vi "get columns.vi"(9 "columns  INFO":string[](array[string]), 10 "columns外部输入":T1, 11 "数组":variant[][](array[variant])) -> (2 "columns output":string[](array[string]), 3 "data":string[][](array[string]))   [LabVIEW 2016, in "SQLite Lib.lvlib"]
uses:
  SQLite Lib.lvlib
  <vilib>/Utility/VariantDataType/VariantType.lvlib
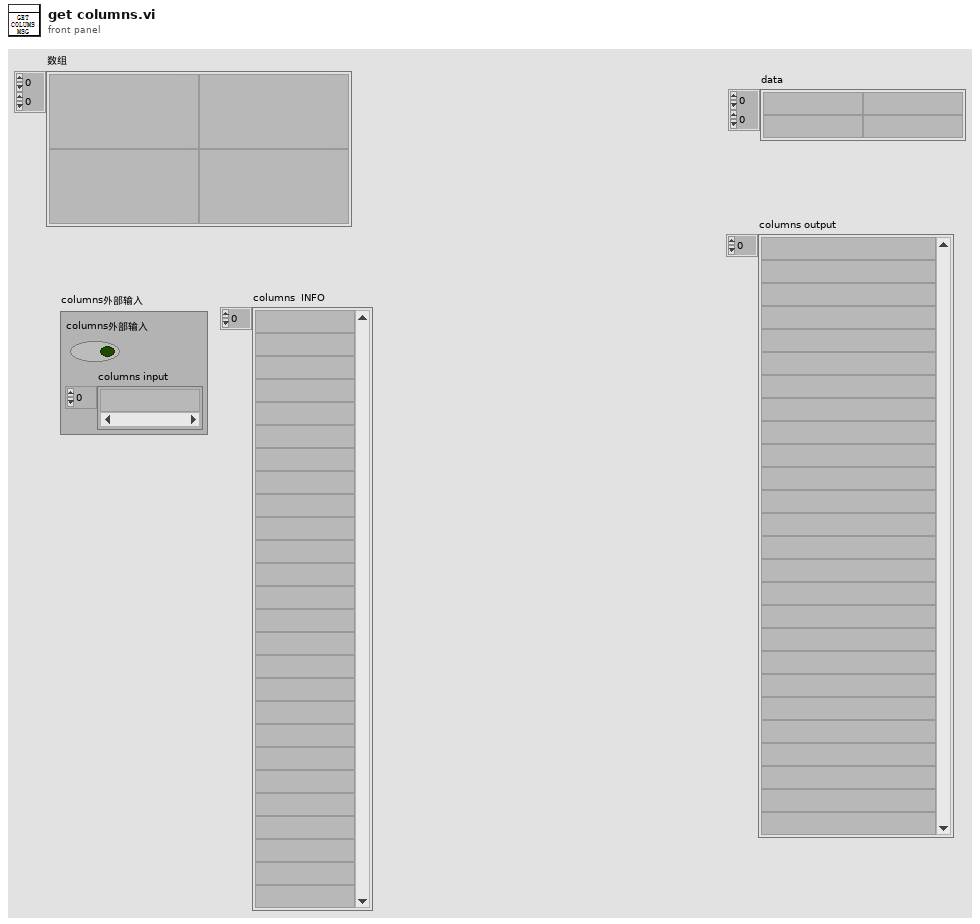
[diagram p1: front panel]
types:
  T1 = cluster{"columns外部输入":bool, "columns input":string[]}
  T2 = typedef "VariantType.lvlib/Type.ctl" = enum8{"Invalid Type", "Void", "I8", "I16", "I32", "I64", "U8", "U16", "U32", "U64", "Single Float", "Double Float", "Extended Float", "Single Complex", "Double Complex", "Extended Complex", "Enum U8", "Enum U16", "Enum U32", "Enum U64", "Single Float With Unit", "Double Float With Unit", "Extended Float With Unit", "Single Complex with Unit", "Double Complex with Unit", "Extended Complex with Unit", "Boolean", "String", "Path", "Picture", "Tag", "Array", "Cluster", "Variant", "LV Variant", "Waveform", "Timestamp", "Digital Waveform", "Digital Data", "ExpressData", "Refnum", "External Data", "VI", "Poly VI", "LabVIEW Class Instance", "Fixed Point"}
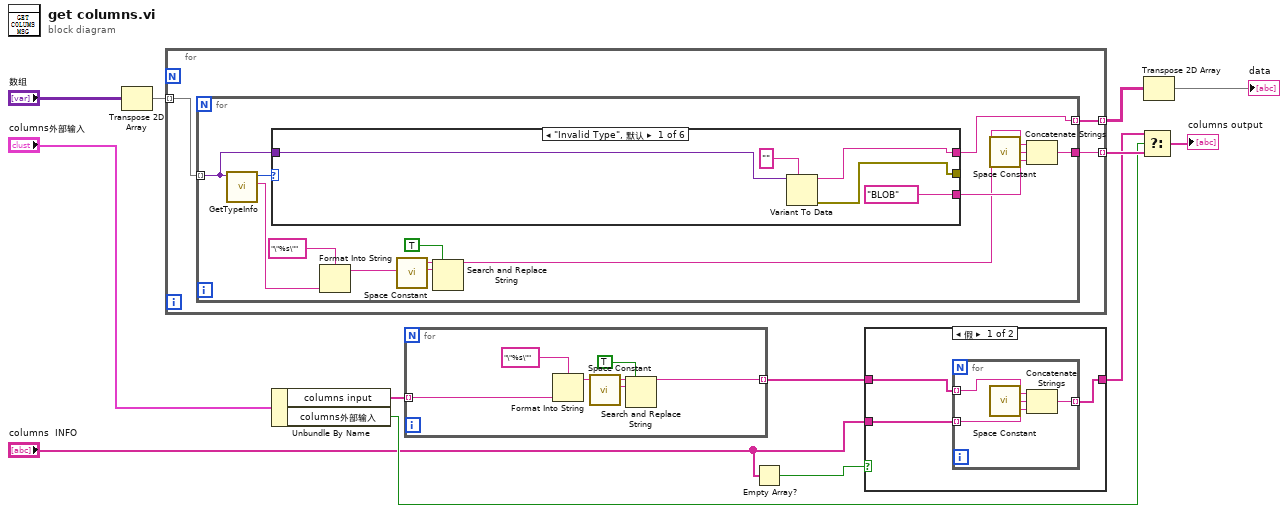
[diagram p0: block diagram]
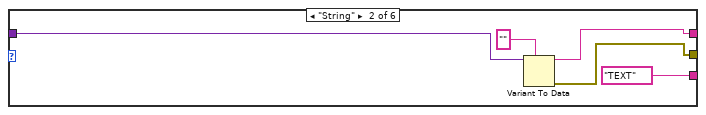
[diagram p3: hidden frame]
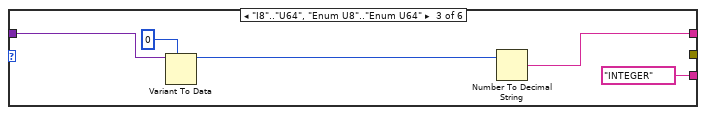
[diagram p4: hidden frame]
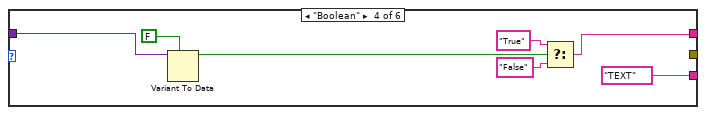
[diagram p5: hidden frame]
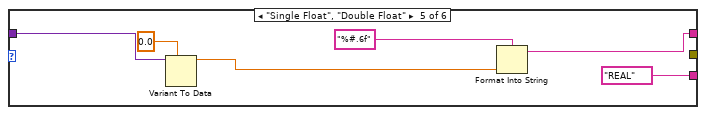
[diagram p6: hidden frame]
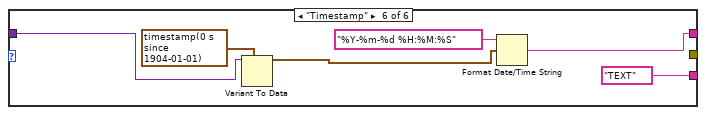
[diagram p7: hidden frame]
diagram:
  n1 = Transpose 2D Array(2D array="数组") -> (transposed array=w11:variant[][])
  n2 = for {
    tunnel: [w14] -> w9 mode=indexing
    tunnel: [w16] -> w12 mode=indexing
    tunnel: w11 -> [w15] mode=indexing
    n3 = for {
      tunnel: [w28] -> w16 mode=indexing
      tunnel: w15 -> [w27] mode=indexing
      tunnel: [w26] -> w14
      n4 = call <vilib>:"GetTypeInfo.vi"("Variant"=w27) -> ("Name"=w21:string, "Type Enum"=w23:T2)  [unwired: 6 in, 3 out]
      n5 = case shown="\"Invalid Type\", 默认" w23 {
        tunnel: w27 -> [w33 w38 w43 w50 w56 w62]
        tunnel: [w31 w36 w40 w44 w53 w59] -> w28
        tunnel: [w30 w35 _ _ _ _] -> _
        tunnel: ["BLOB" ("组合框") "TEXT" ("组合框") "INTEGER" ("组合框") "TEXT" ("组合框") "REAL" ("组合框") "TEXT" ("组合框")] -> w25
        frame "Invalid Type", Default {
          n6 = Variant To Data(type="", Variant=w33) -> (data=w31:string, error out=w30:errorcluster)  [unwired: 1 in]
        }
        frame "String" {
          n7 = Variant To Data(type="", Variant=w38) -> (data=w36:string, error out=w35:errorcluster)  [unwired: 1 in]
        }
        frame "I8".."U64", "Enum U8".."Enum U64" {
          n8 = Variant To Data(type=0, Variant=w43) -> (data=w41:i32)  [unwired: 1 in, 1 out]
          n9 = Number To Decimal String(number=w41) -> (decimal integer string=w40:string)  [unwired: 1 in]
        }
        frame "Boolean" {
          n10 = Variant To Data(type=FALSE, Variant=w50) -> (data=w47:bool)  [unwired: 1 in, 1 out]
          n11 = Select(t="True", s=w47, f="False") -> (s? t:f=w44:string)
        }
        frame "Single Float", "Double Float" {
          n12 = Variant To Data(type=sgl 0.0, Variant=w56) -> (data=w54:sgl)  [unwired: 1 in, 1 out]
          n13 = Format Into String(format string="%#.6f" ("格式字符串"), w54) -> (resulting string=w53:string)  [unwired: 2 in, 1 out]
        }
        frame "Timestamp" {
          n14 = Variant To Data(type=timestamp(0 s since 1904-01-01) ("时间标识"), Variant=w62) -> (data=w60:timestamp)  [unwired: 1 in, 1 out]
          n15 = Format Date/Time String(time format string (%c)="%Y-%m-%d %H:%M:%S" ("时间格式字符串(%c)"), seconds (now)=w60) -> (date/time string=w59:string)  [unwired: 1 in]
        }
      }
      n16 = Format Into String(format string="\"%s\"" ("格式字符串"), w21) -> (resulting string=w20:string)  [unwired: 2 in, 1 out]
      n17 = call <vilib>:"Space Constant.vi"() -> ("String"=w18:string)
      n18 = Search and Replace String(replace all?=TRUE ("替换全部？(F)"), input string=w20, search string=w18) -> (result string=w19:string)  [unwired: 5 in, 3 out]
      n19 = call <vilib>:"Space Constant.vi"() -> ("String"=w24:string)
      n20 = Concatenate Strings(w19, w24, w25) -> (w26:string)
    }
  }
  n21 = Unbundle By Name("columns外部输入") -> ("columns input"=w5:string[], "columns外部输入"=w6:bool)
  n22 = for {
    tunnel: w5 -> [w68] mode=indexing
    tunnel: [w63] -> w4 mode=indexing
    n23 = Format Into String(format string="\"%s\"" ("格式字符串"), w68) -> (resulting string=w64:string)  [unwired: 2 in, 1 out]
    n24 = call <vilib>:"Space Constant.vi"() -> ("String"=w66:string)
    n25 = Search and Replace String(replace all?=TRUE ("替换全部？(F)"), input string=w64, search string=w66) -> (result string=w63:string)  [unwired: 5 in, 3 out]
  }
  n26 = Empty Array?(array="columns  INFO") -> (empty?=w1:bool)
  n27 = case shown="假" w1 {
    tunnel: w4 -> [w71 w76]
    tunnel: [w70 w76] -> w3
    tunnel: "columns  INFO" -> [w69 _]
    frame False {
      n28 = for {
        tunnel: w71 -> [w74] mode=indexing
        tunnel: w69 -> [w73] mode=indexing
        tunnel: [w72] -> w70 mode=indexing
        n29 = call <vilib>:"Space Constant.vi"() -> ("String"=w75:string)
        n30 = Concatenate Strings(w74, w75, w73) -> (w72:string)
      }
    }
    frame True {
    }
  }
  n31 = Select(t=w3, s=w6, f=w9) -> (s? t:f=→"columns output":string[])
  n32 = Transpose 2D Array(2D array=w12) -> (transposed array=→"data":string[][])
